vi "Inspect HDI Pad Groups.vi"(8 "error in":errorcluster, 9 "Slot":i32, 10 "Chuck":i32, 11 "Potting Procedure in":refnum<class "Potting Procedure.lvclass">) -> (0 "error out":errorcluster, 3 "Potting Procedure out":refnum<class "Potting Procedure.lvclass">)   [LabVIEW 2011, in "Potting Procedure.lvclass"]
uses:
  Potting Procedure.lvclass
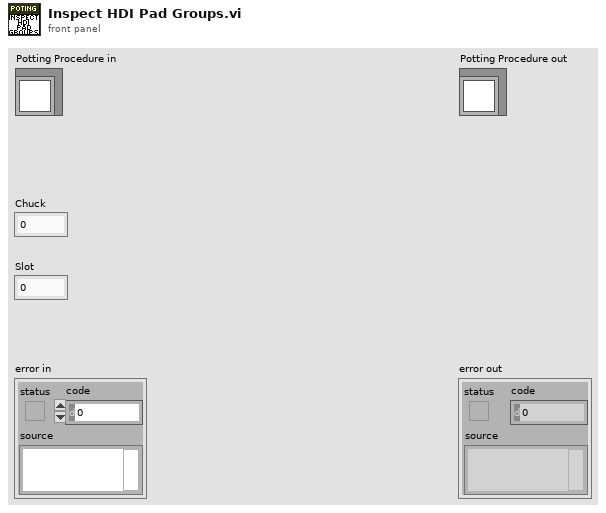
[diagram p1: front panel]
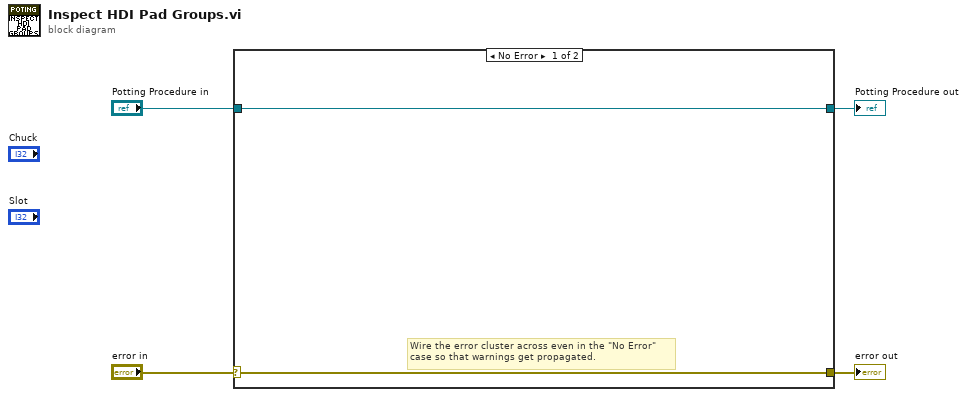
[diagram p0: block diagram]
diagram:
  n1 = case shown="No Error" "error in" {
    selector: "error in" -> [w5 w8]
    tunnel: [w5 w8] -> w3
    tunnel: [w6 w7] -> w1
    tunnel: "Potting Procedure in" -> [w6 w7]
    frame No Error {
      # "Wire the error cluster across even in the \"No Error\"\ncase so that warnings get propagated."
    }
    frame Error {
    }
  }
  "error out" <- w3
  "Potting Procedure out" <- w1
